vi "Send Start Measurements.vi"(4 "Objects enqueuers":refnum<class "Message Enqueuer.lvclass">[](array[class]), 6 "Reply to":refnum<class "Result Reply Msg.lvclass">, 7 "Message Priority (Normal)":T1=enum."Normal", 8 "error in (no error)":errorcluster, 9 "Repeat times":i32=1, 10 "Objects":string[](array[string]), 11 "Message Enqueuer":refnum<class "Message Enqueuer.lvclass">) -> (0 "error out":errorcluster, 3 "Message Enqueuer out":refnum<class "Message Enqueuer.lvclass">)   [LabVIEW 2015, in "Start Measurements Msg.lvclass"]
doc: "This VI sends the message to an actor."
uses:
  Start Measurements Msg.lvclass
  <vilib>/ActorFramework/Message Enqueuer/Message Enqueuer.lvclass
  <vilib>/ActorFramework/Message Enqueuer/Message Priority.ctl
  Measure Object Messages/Result Reply Msg/Result Reply Msg.lvclass
  Start Measurements Msg.lvclass/Start Measurements Msg.ctl
  <vilib>/ActorFramework/Message Enqueuer/Message Enqueuer.lvclass/Message Enqueuer.ctl
  <vilib>/ActorFramework/Message Priority Queue/Priority Enqueue.vi
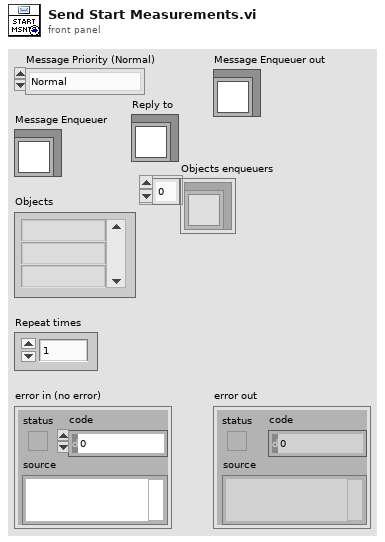
[diagram p1: front panel]
types:
  T1 = typedef "Actor Framework.lvlib/Message Enqueuer.lvclass/Message Priority.ctl" = enum16{"Low", "Normal", "High"}
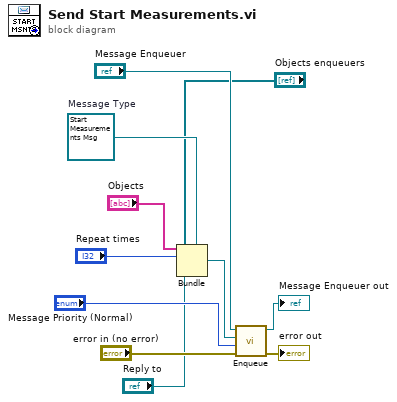
[diagram p0: block diagram]
diagram:
  w8 = refnum<class "Start Measurements Msg.lvclass"> refnum  # Message Type
  n1 = Bundle(cluster=w8, "Objects", "Repeat times", "Reply to", "Objects enqueuers") -> (w7:refnum<class "Start Measurements Msg.lvclass">)
  n2 = call <vilib>:"Enqueue.vi"("error in (no error)"="error in (no error)", "Message Priority (Normal)"="Message Priority (Normal)", "Message"=w7, "Message Enqueuer in"="Message Enqueuer") -> ("error out"=→"error out":errorcluster, "Message Enqueuer out"=→"Message Enqueuer out":refnum<class "Message Enqueuer.lvclass">)  [unwired: 6 in]
